vi "Day02-02.vi"() -> ()   [LabVIEW 2021]
panel:
  out "타임 아웃":dbl
  in  "정지 정지 정지 2":bool
  in  "확인 확인 확인 2":bool
  in  "정지 정지 정지":bool
  in  "확인 확인 확인":bool
  out "결과":dbl
  in  "숫자형 2":dbl
  in  "숫자형":dbl
  out "케이스를 지난 출력 결과":i32
  # "< 열거형 케이스 구조 >"
  # "< 이벤트 구조 >"
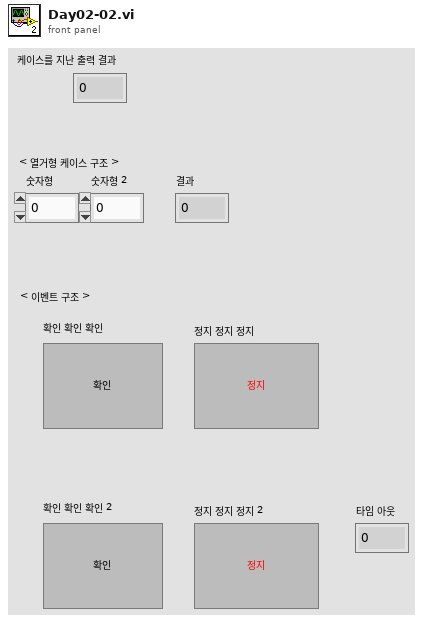
[diagram p1: front panel]
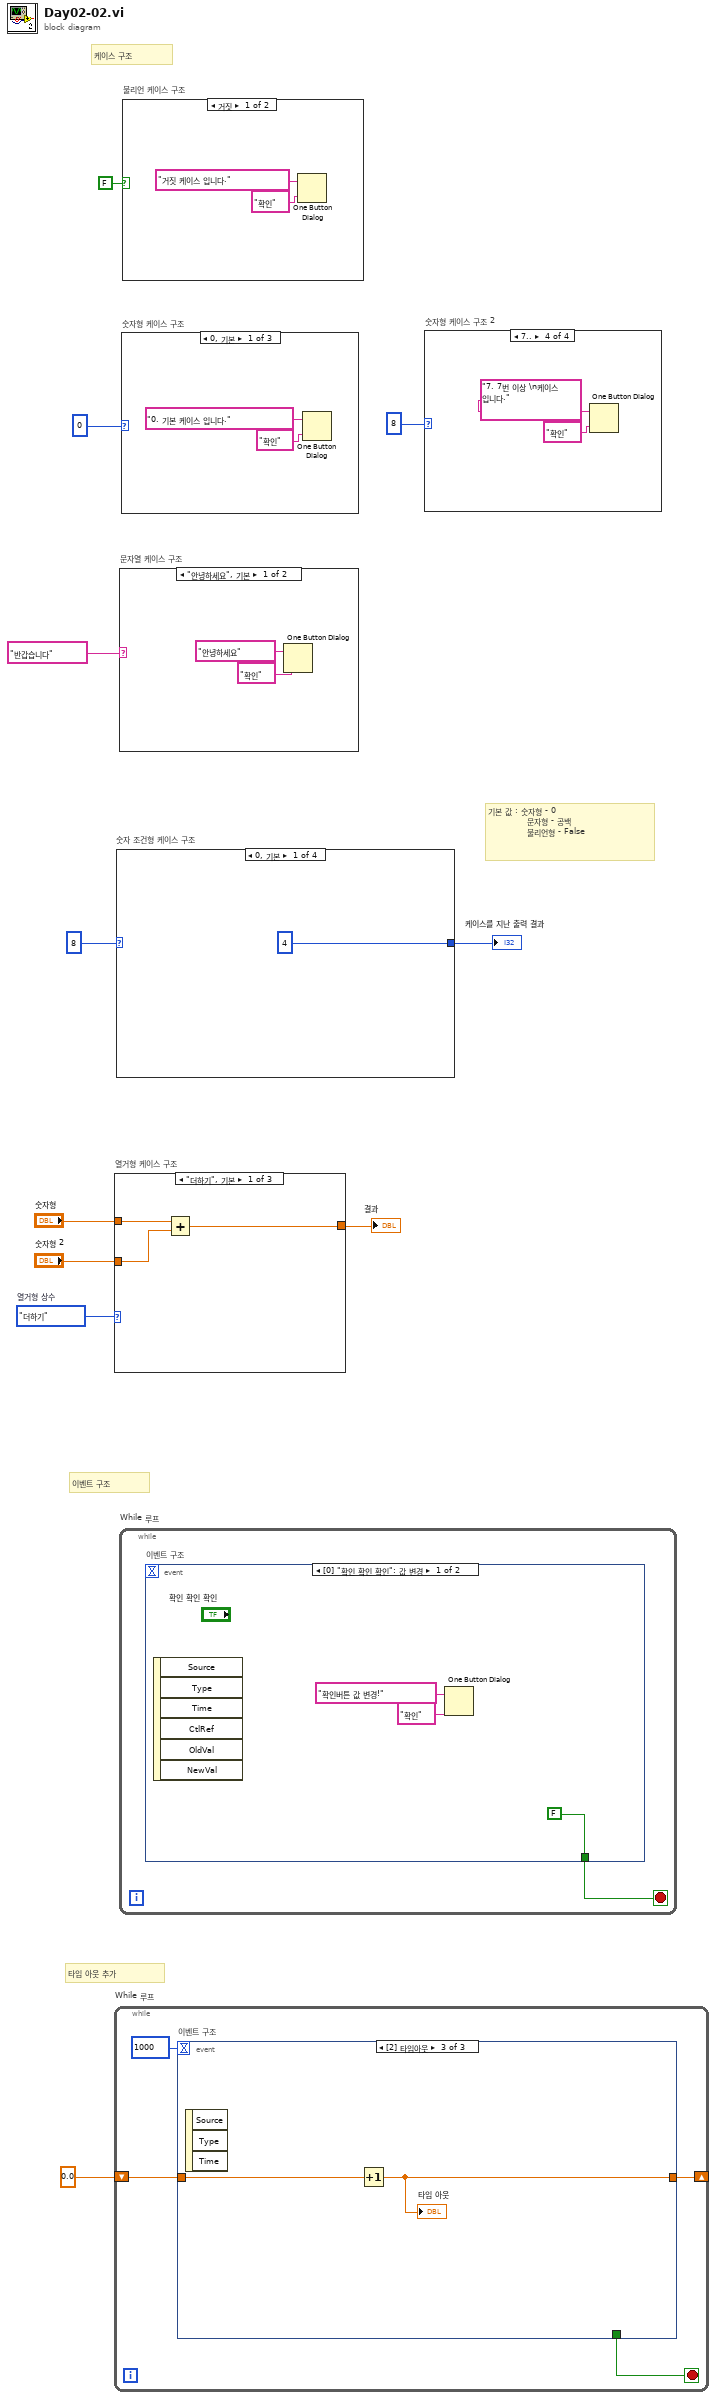
[diagram p0: block diagram]
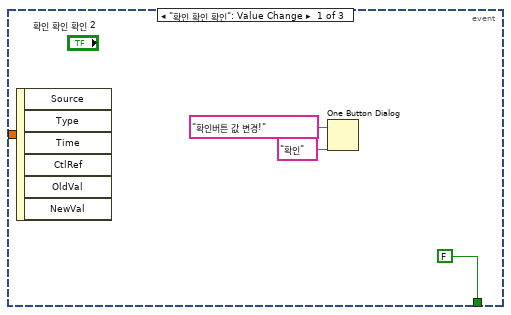
[diagram p2: hidden frame]
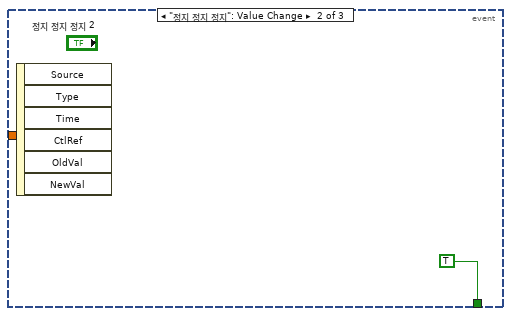
[diagram p3: hidden frame]
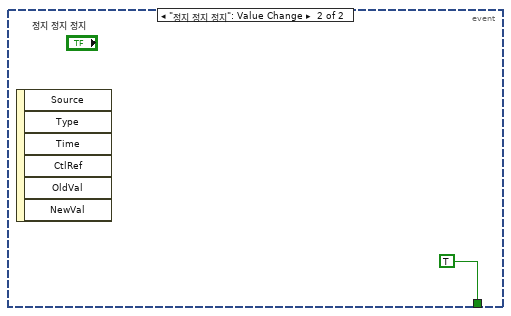
[diagram p4: hidden frame]
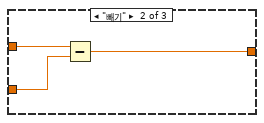
[diagram p5: hidden frame]
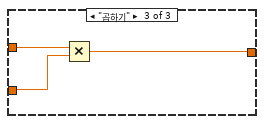
[diagram p6: hidden frame]
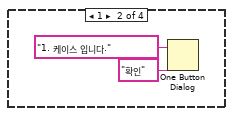
[diagram p7: hidden frame]
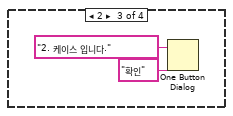
[diagram p8: hidden frame]
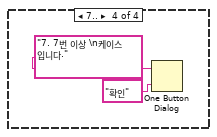
[diagram p9: hidden frame]
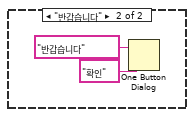
[diagram p10: hidden frame]
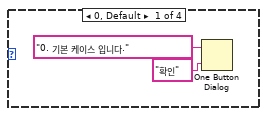
[diagram p11: hidden frame]
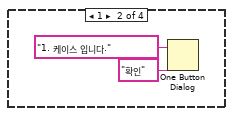
[diagram p12: hidden frame]
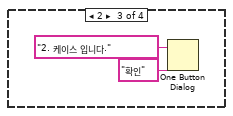
[diagram p13: hidden frame]
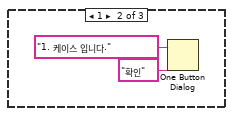
[diagram p14: hidden frame]
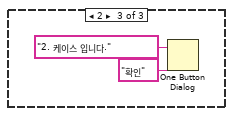
[diagram p15: hidden frame]
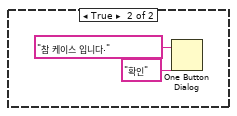
[diagram p16: hidden frame]
diagram:
  w5 = enum16{"더하기", "빼기", "곱하기"}."더하기"  # 열거형 상수
  # "타임 아웃 추가"
  # "이벤트 구조"
  # "기본 값 : 숫자형 - 0\n             문자형 - 공백\n             불리언형 - False"
  # "케이스 구조"
  n1 = case "열거형 케이스 구조" shown="\"더하기\", 기본" w5 {
    tunnel: "숫자형" -> [w14 w17 w20]
    tunnel: "숫자형 2" -> [w13 w16 w19]
    tunnel: [w12 w15 w18] -> w2
    frame "더하기", Default {
      n2 = Add(x=w14, y=w13) -> (x+y=w12:dbl)
    }
    frame "빼기" {
      n3 = Subtract(x=w17, y=w16) -> (x-y=w15:dbl)
    }
    frame "곱하기" {
      n4 = Multiply(x=w20, y=w19) -> (x*y=w18:dbl)
    }
  }
  "결과" <- w2
  n5 = while "While 루프" {
    shift-right: [w21] -> _
    shift-left: 0.0 -> [w22]
    stop <- w24 stop-if-true
    n6 = event "이벤트 구조" shown="[2] 타임아웃" {
      selector: _ -> [_ _ _]
      dyn-events: _ -> [_ _ _]
      timeout: 1000 -> [_ _ _]
      tunnel: [FALSE TRUE _] -> w24
      tunnel: w22 -> [_ _ w30]
      tunnel: [_ _ w29] -> w21
      event "확인 확인 확인": Value Change {
        n7 = event-data() -> ()  [unwired: 1 in, 6 out]
        n8 = One Button Dialog(message="확인버튼 값 변경!" ("메시지"), button name ("OK")="확인" ("버튼 이름(\"확인\")")) -> ()  [unwired: 1 out]
      }
      event "정지 정지 정지": Value Change {
        n9 = event-data() -> ()  [unwired: 1 in, 6 out]
      }
      event Timeout {
        n10 = event-data() -> ()  [unwired: 1 in, 3 out]
        n11 = Increment(x=w30) -> (x+1=w29:dbl)
        "타임 아웃" <- w29
      }
    }
  }
  n12 = case "숫자 조건형 케이스 구조" shown="0, 기본" 8 {
    tunnel: [4 _ _ _] -> w6
    frame 0, Default {
    }
    frame 1 {
      n13 = One Button Dialog(message="1. 케이스 입니다." ("메시지"), button name ("OK")="확인" ("버튼 이름(\"확인\")")) -> ()  [unwired: 1 out]
    }
    frame 2 {
      n14 = One Button Dialog(message="2. 케이스 입니다." ("메시지"), button name ("OK")="확인" ("버튼 이름(\"확인\")")) -> ()  [unwired: 1 out]
    }
    frame 7.. {
      n15 = One Button Dialog(message="7. 7번 이상 \n케이스 입니다." ("메시지"), button name ("OK")="확인" ("버튼 이름(\"확인\")")) -> ()  [unwired: 1 out]
    }
  }
  "케이스를 지난 출력 결과" <- w6
  n16 = case "문자열 케이스 구조" shown="\"안녕하세요\", 기본" "반갑습니다" {
    frame "안녕하세요", Default {
      n17 = One Button Dialog(message="안녕하세요" ("메시지"), button name ("OK")="확인" ("버튼 이름(\"확인\")")) -> ()  [unwired: 1 out]
    }
    frame "반갑습니다" {
      n18 = One Button Dialog(message="반갑습니다" ("메시지"), button name ("OK")="확인" ("버튼 이름(\"확인\")")) -> ()  [unwired: 1 out]
    }
  }
  n19 = while "While 루프" {
    stop <- w42 stop-if-true
    n20 = event "이벤트 구조" shown="[0] \"확인 확인 확인\": 값 변경" {
      selector: _ -> [_ _]
      dyn-events: _ -> [_ _]
      timeout: _ -> [_ _]
      tunnel: [FALSE TRUE] -> w42
      event "확인 확인 확인": Value Change {
        n21 = event-data() -> ()  [unwired: 1 in, 6 out]
        n22 = One Button Dialog(message="확인버튼 값 변경!" ("메시지"), button name ("OK")="확인" ("버튼 이름(\"확인\")")) -> ()  [unwired: 1 out]
      }
      event "정지 정지 정지": Value Change {
        n23 = event-data() -> ()  [unwired: 1 in, 6 out]
      }
    }
  }
  n24 = case "숫자형 케이스 구조" shown="0, 기본" 0 {
    frame 0, Default {
      n25 = One Button Dialog(message="0. 기본 케이스 입니다." ("메시지"), button name ("OK")="확인" ("버튼 이름(\"확인\")")) -> ()  [unwired: 1 out]
    }
    frame 1 {
      n26 = One Button Dialog(message="1. 케이스 입니다." ("메시지"), button name ("OK")="확인" ("버튼 이름(\"확인\")")) -> ()  [unwired: 1 out]
    }
    frame 2 {
      n27 = One Button Dialog(message="2. 케이스 입니다." ("메시지"), button name ("OK")="확인" ("버튼 이름(\"확인\")")) -> ()  [unwired: 1 out]
    }
  }
  n28 = case "불리언 케이스 구조" shown="거짓" FALSE {
    frame False {
      n29 = One Button Dialog(message="거짓 케이스 입니다." ("메시지"), button name ("OK")="확인" ("버튼 이름(\"확인\")")) -> ()  [unwired: 1 out]
    }
    frame True {
      n30 = One Button Dialog(message="참 케이스 입니다." ("메시지"), button name ("OK")="확인" ("버튼 이름(\"확인\")")) -> ()  [unwired: 1 out]
    }
  }
  n31 = case "숫자형 케이스 구조 2" shown="7.." 8 {
    frame 0, Default {
      n32 = One Button Dialog(message="0. 기본 케이스 입니다." ("메시지"), button name ("OK")="확인" ("버튼 이름(\"확인\")")) -> ()  [unwired: 1 out]
    }
    frame 1 {
      n33 = One Button Dialog(message="1. 케이스 입니다." ("메시지"), button name ("OK")="확인" ("버튼 이름(\"확인\")")) -> ()  [unwired: 1 out]
    }
    frame 2 {
      n34 = One Button Dialog(message="2. 케이스 입니다." ("메시지"), button name ("OK")="확인" ("버튼 이름(\"확인\")")) -> ()  [unwired: 1 out]
    }
    frame 7.. {
      n35 = One Button Dialog(message="7. 7번 이상 \n케이스 입니다." ("메시지"), button name ("OK")="확인" ("버튼 이름(\"확인\")")) -> ()  [unwired: 1 out]
    }
  }
